vi "duplicates.vi"(11 "Array":string[](array[string])=["a", "b", "f", "e", "d"]) -> (3 "Array 2":string[](array[string]))   [LabVIEW 2014]
uses:
  Alphabet.ctl
  Counting.ctl
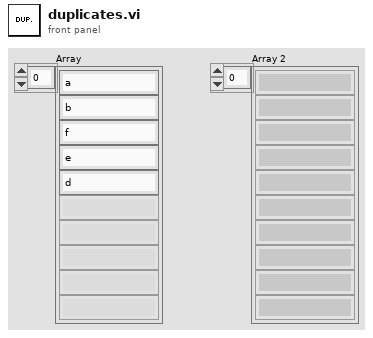
[diagram p1: front panel]
types:
  T1 = typedef "Counting.ctl" = cluster{"list":i32[], "a":i32}
  T2 = typedef "Alphabet.ctl" = enum16{"a", "b", "c", "d", "e", "f", "g", "h", "i", "j", "k", "l", "m", "n", "o", "p", "q", "r", "s", "t", "u", "v", "x", "y", "w", "z", "output"}
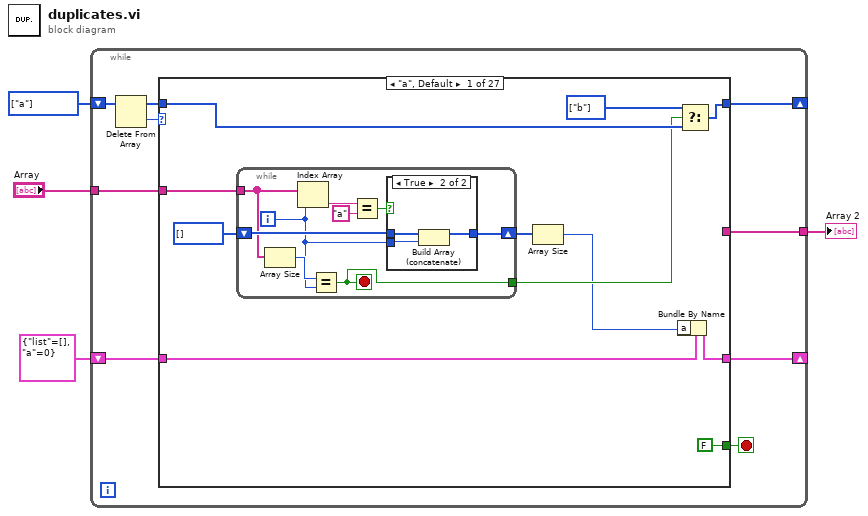
[diagram p0: block diagram]
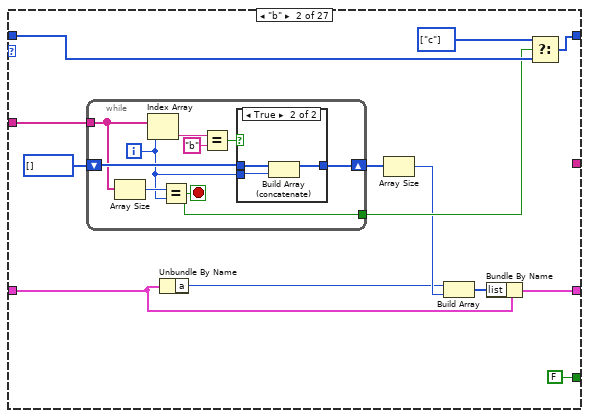
[diagram p3: hidden frame]
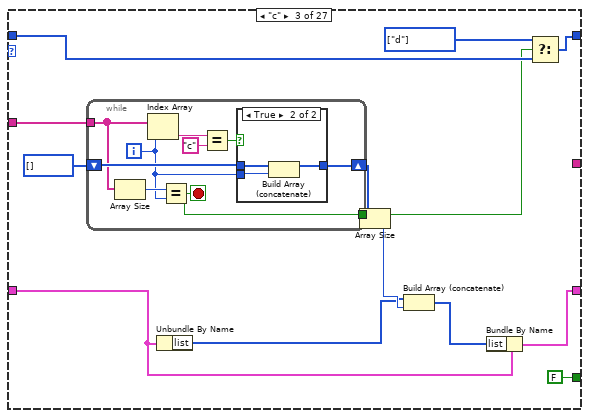
[diagram p5: hidden frame]
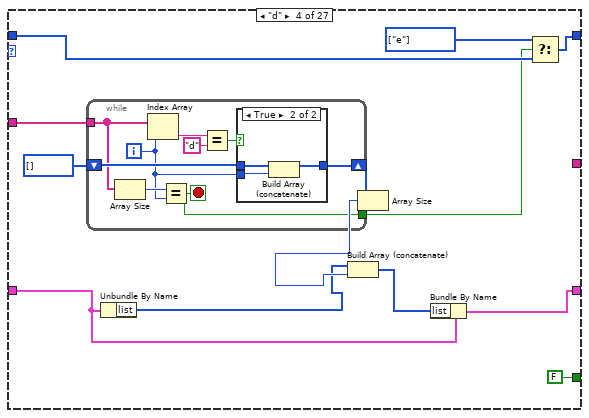
[diagram p7: hidden frame]
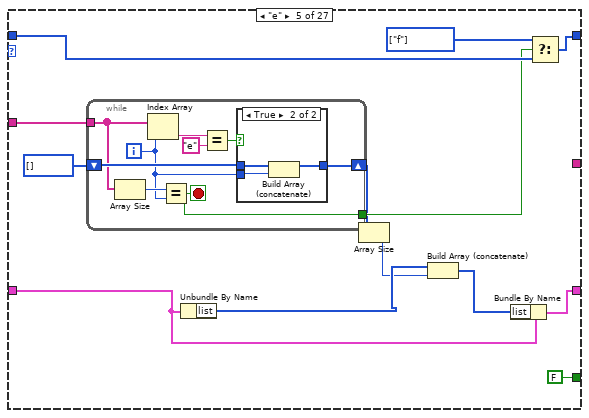
[diagram p9: hidden frame]
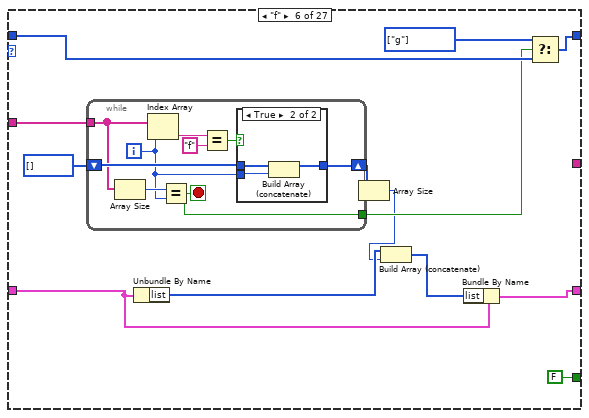
[diagram p11: hidden frame]
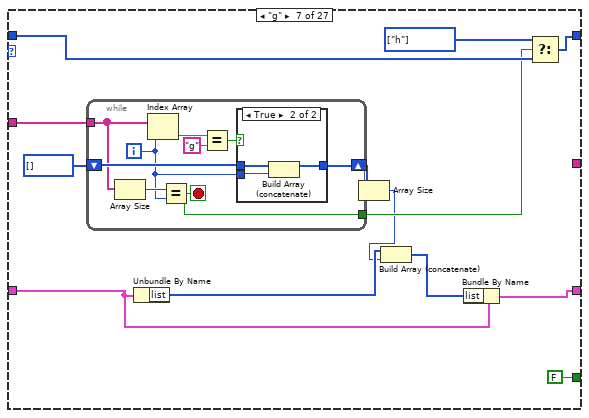
[diagram p13: hidden frame]
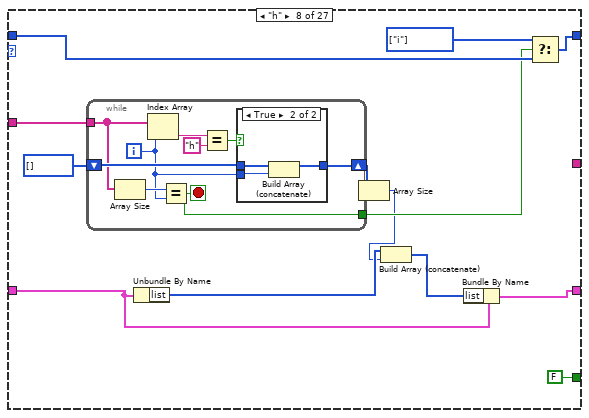
[diagram p15: hidden frame]
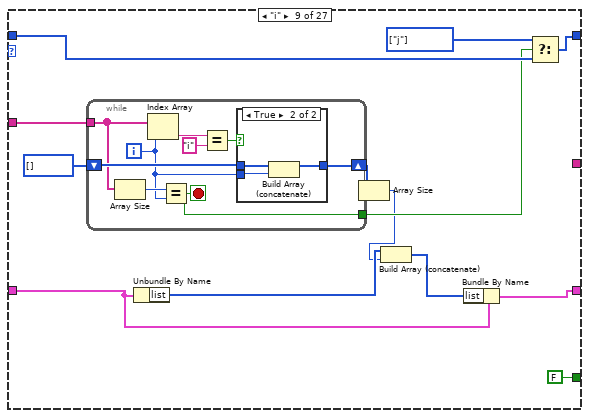
[diagram p17: hidden frame]
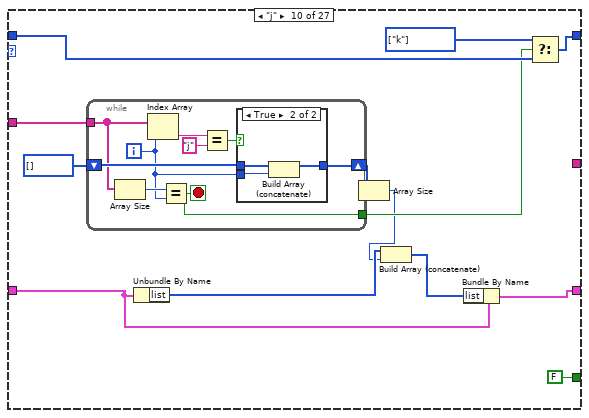
[diagram p19: hidden frame]
diagram:
  w4 = T2[] [enum."a"] items=["a", "b", "c", "d", "e", "f", "g", "h", "i", "j", "k", "l", "m", "n", "o", "p", "q", "r", "s", "t", "u", "v", "x", "y", "w", "z", "output"]
  n1 = while {
    shift-right: [w11] -> _
    shift-left: w4 -> [w13]
    tunnel: "Array" -> [w9]
    shift-right: [w6] -> _
    shift-left: T1 {"list"=[], "a"=0} -> [w7]
    tunnel: [w5] -> w1
    stop <- w8 stop-if-true
    n2 = Delete From Array(array=w13) -> (deleted portion=w12:T2, array with subset deleted=w10:T2[])  [unwired: 2 in]
    n3 = case shown="\"a\", Default" w12 {
      tunnel: [w21 w47 w73 w99 w125 w151 w177 w203 w229 w255 w281 w307 w333 w359 w385 w411 w437 w463 w489 w515 w541 w567 w593 w619 w645 w671 w690] -> w11
      tunnel: w10 -> [w23 w49 w75 w101 w127 w153 w179 w205 w231 w257 w283 w309 w335 w361 w387 w413 w439 w465 w491 w517 w543 w569 w595 w621 w647 w673 w690]
      tunnel: w9 -> [w24 w50 w76 w102 w128 w154 w180 w206 w232 w258 w284 w310 w336 w362 w388 w414 w440 w466 w492 w518 w544 w570 w596 w622 w648 w674 _]
      tunnel: [FALSE FALSE FALSE FALSE FALSE FALSE FALSE FALSE FALSE FALSE FALSE FALSE FALSE FALSE FALSE FALSE FALSE FALSE FALSE FALSE FALSE FALSE FALSE FALSE FALSE FALSE TRUE] -> w8
      tunnel: w7 -> [w16 w42 w68 w94 w118 w144 w170 w196 w222 w248 w274 w300 w326 w352 w378 w404 w430 w456 w482 w508 w534 w560 w586 w612 w638 w664 w692]
      tunnel: [w15 w41 w67 w93 w119 w145 w171 w197 w223 w249 w275 w301 w327 w353 w379 w405 w431 w457 w483 w509 w535 w561 w587 w613 w639 w665 w692] -> w6
      tunnel: [_ _ _ _ _ _ _ _ _ _ _ _ _ _ _ _ _ _ _ _ _ _ _ _ _ _ w688] -> w5
      frame "a", Default {
        w22 = T2[] [enum."b"] items=["a", "b", "c", "d", "e", "f", "g", "h", "i", "j", "k", "l", "m", "n", "o", "p", "q", "r", "s", "t", "u", "v", "x", "y", "w", "z", "output"]
        n4 = while {
          tunnel: w24 -> [w28]
          shift-right: [w29] -> w17
          shift-left: i32[] [] -> [w30]
          tunnel: [w25] -> w18
          i -> [w26]
          stop <- w25 stop-if-true
          n5 = Array Size(array=w28) -> (size(s)=w27:i32)
          n6 = Index Array(array=w28, index=w26) -> (element=w31:string)
          n7 = Equal?(x=w27, y=w26) -> (x = y?=w25:bool)
          n8 = Equal?(x=w31, y="a") -> (x = y?=w32:bool)
          n9 = case shown="True" w32 {
            tunnel: w26 -> [_ w37]
            tunnel: w30 -> [w34 w36]
            tunnel: [w34 w35] -> w29
            frame False {
            }
            frame True {
              n10 = Build Array (concatenate)(w36, w37) -> (w35:i32[])
            }
          }
        }
        n11 = Array Size(array=w17) -> (size(s)=w14:i32)
        n12 = Bundle By Name(cluster=w16, "a"=w14) -> (w15:T1)
        n13 = Select(t=w22, s=w18, f=w23) -> (s? t:f=w21:T2[])
      }
      frame "b" {
        w48 = T2[] [enum."c"] items=["a", "b", "c", "d", "e", "f", "g", "h", "i", "j", "k", "l", "m", "n", "o", "p", "q", "r", "s", "t", "u", "v", "x", "y", "w", "z", "output"]
        n14 = while {
          tunnel: w50 -> [w54]
          shift-right: [w55] -> w43
          shift-left: i32[] [] -> [w56]
          tunnel: [w51] -> w44
          i -> [w52]
          stop <- w51 stop-if-true
          n15 = Array Size(array=w54) -> (size(s)=w53:i32)
          n16 = Index Array(array=w54, index=w52) -> (element=w57:string)
          n17 = Equal?(x=w53, y=w52) -> (x = y?=w51:bool)
          n18 = Equal?(x=w57, y="b") -> (x = y?=w58:bool)
          n19 = case shown="True" w58 {
            tunnel: w52 -> [_ w63]
            tunnel: w56 -> [w60 w62]
            tunnel: [w60 w61] -> w55
            frame False {
            }
            frame True {
              n20 = Build Array (concatenate)(w62, w63) -> (w61:i32[])
            }
          }
        }
        n21 = Unbundle By Name(w42) -> ("a"=w38:i32)
        n22 = Array Size(array=w43) -> (size(s)=w39:i32)
        n23 = Build Array(w38, w39) -> (w40:i32[])
        n24 = Bundle By Name(cluster=w42, "list"=w40) -> (w41:T1)
        n25 = Select(t=w48, s=w44, f=w49) -> (s? t:f=w47:T2[])
      }
      frame "c" {
        w74 = T2[] [enum."d"] items=["a", "b", "c", "d", "e", "f", "g", "h", "i", "j", "k", "l", "m", "n", "o", "p", "q", "r", "s", "t", "u", "v", "x", "y", "w", "z", "output"]
        n26 = while {
          tunnel: w76 -> [w80]
          shift-right: [w81] -> w66
          shift-left: i32[] [] -> [w82]
          tunnel: [w77] -> w70
          i -> [w78]
          stop <- w77 stop-if-true
          n27 = Array Size(array=w80) -> (size(s)=w79:i32)
          n28 = Index Array(array=w80, index=w78) -> (element=w83:string)
          n29 = Equal?(x=w79, y=w78) -> (x = y?=w77:bool)
          n30 = Equal?(x=w83, y="c") -> (x = y?=w84:bool)
          n31 = case shown="True" w84 {
            tunnel: w78 -> [_ w89]
            tunnel: w82 -> [w86 w88]
            tunnel: [w86 w87] -> w81
            frame False {
            }
            frame True {
              n32 = Build Array (concatenate)(w88, w89) -> (w87:i32[])
            }
          }
        }
        n33 = Unbundle By Name(w68) -> ("list"=w64:i32[])
        n34 = Array Size(array=w66) -> (size(s)=w65:i32)
        n35 = Build Array (concatenate)(w64, w65) -> (w69:i32[])
        n36 = Bundle By Name(cluster=w68, "list"=w69) -> (w67:T1)
        n37 = Select(t=w74, s=w70, f=w75) -> (s? t:f=w73:T2[])
      }
      frame "d" {
        w100 = T2[] [enum."e"] items=["a", "b", "c", "d", "e", "f", "g", "h", "i", "j", "k", "l", "m", "n", "o", "p", "q", "r", "s", "t", "u", "v", "x", "y", "w", "z", "output"]
        n38 = while {
          tunnel: w102 -> [w106]
          shift-right: [w107] -> w92
          shift-left: i32[] [] -> [w108]
          tunnel: [w103] -> w96
          i -> [w104]
          stop <- w103 stop-if-true
          n39 = Array Size(array=w106) -> (size(s)=w105:i32)
          n40 = Index Array(array=w106, index=w104) -> (element=w109:string)
          n41 = Equal?(x=w105, y=w104) -> (x = y?=w103:bool)
          n42 = Equal?(x=w109, y="d") -> (x = y?=w110:bool)
          n43 = case shown="True" w110 {
            tunnel: w104 -> [_ w115]
            tunnel: w108 -> [w112 w114]
            tunnel: [w112 w113] -> w107
            frame False {
            }
            frame True {
              n44 = Build Array (concatenate)(w114, w115) -> (w113:i32[])
            }
          }
        }
        n45 = Unbundle By Name(w94) -> ("list"=w90:i32[])
        n46 = Array Size(array=w92) -> (size(s)=w91:i32)
        n47 = Build Array (concatenate)(w90, w91) -> (w95:i32[])
        n48 = Bundle By Name(cluster=w94, "list"=w95) -> (w93:T1)
        n49 = Select(t=w100, s=w96, f=w101) -> (s? t:f=w99:T2[])
      }
      frame "e" {
        w126 = T2[] [enum."f"] items=["a", "b", "c", "d", "e", "f", "g", "h", "i", "j", "k", "l", "m", "n", "o", "p", "q", "r", "s", "t", "u", "v", "x", "y", "w", "z", "output"]
        n50 = while {
          tunnel: w128 -> [w132]
          shift-right: [w133] -> w120
          shift-left: i32[] [] -> [w134]
          tunnel: [w129] -> w122
          i -> [w130]
          stop <- w129 stop-if-true
          n51 = Array Size(array=w132) -> (size(s)=w131:i32)
          n52 = Index Array(array=w132, index=w130) -> (element=w135:string)
          n53 = Equal?(x=w131, y=w130) -> (x = y?=w129:bool)
          n54 = Equal?(x=w135, y="e") -> (x = y?=w136:bool)
          n55 = case shown="True" w136 {
            tunnel: w130 -> [_ w141]
            tunnel: w134 -> [w138 w140]
            tunnel: [w138 w139] -> w133
            frame False {
            }
            frame True {
              n56 = Build Array (concatenate)(w140, w141) -> (w139:i32[])
            }
          }
        }
        n57 = Unbundle By Name(w118) -> ("list"=w117:i32[])
        n58 = Array Size(array=w120) -> (size(s)=w116:i32)
        n59 = Build Array (concatenate)(w117, w116) -> (w121:i32[])
        n60 = Bundle By Name(cluster=w118, "list"=w121) -> (w119:T1)
        n61 = Select(t=w126, s=w122, f=w127) -> (s? t:f=w125:T2[])
      }
      frame "f" {
        w152 = T2[] [enum."g"] items=["a", "b", "c", "d", "e", "f", "g", "h", "i", "j", "k", "l", "m", "n", "o", "p", "q", "r", "s", "t", "u", "v", "x", "y", "w", "z", "output"]
        n62 = while {
          tunnel: w154 -> [w158]
          shift-right: [w159] -> w146
          shift-left: i32[] [] -> [w160]
          tunnel: [w155] -> w148
          i -> [w156]
          stop <- w155 stop-if-true
          n63 = Array Size(array=w158) -> (size(s)=w157:i32)
          n64 = Index Array(array=w158, index=w156) -> (element=w161:string)
          n65 = Equal?(x=w157, y=w156) -> (x = y?=w155:bool)
          n66 = Equal?(x=w161, y="f") -> (x = y?=w162:bool)
          n67 = case shown="True" w162 {
            tunnel: w156 -> [_ w167]
            tunnel: w160 -> [w164 w166]
            tunnel: [w164 w165] -> w159
            frame False {
            }
            frame True {
              n68 = Build Array (concatenate)(w166, w167) -> (w165:i32[])
            }
          }
        }
        n69 = Unbundle By Name(w144) -> ("list"=w143:i32[])
        n70 = Array Size(array=w146) -> (size(s)=w142:i32)
        n71 = Build Array (concatenate)(w143, w142) -> (w147:i32[])
        n72 = Bundle By Name(cluster=w144, "list"=w147) -> (w145:T1)
        n73 = Select(t=w152, s=w148, f=w153) -> (s? t:f=w151:T2[])
      }
      frame "g" {
        w178 = T2[] [enum."h"] items=["a", "b", "c", "d", "e", "f", "g", "h", "i", "j", "k", "l", "m", "n", "o", "p", "q", "r", "s", "t", "u", "v", "x", "y", "w", "z", "output"]
        n74 = while {
          tunnel: w180 -> [w184]
          shift-right: [w185] -> w172
          shift-left: i32[] [] -> [w186]
          tunnel: [w181] -> w174
          i -> [w182]
          stop <- w181 stop-if-true
          n75 = Array Size(array=w184) -> (size(s)=w183:i32)
          n76 = Index Array(array=w184, index=w182) -> (element=w187:string)
          n77 = Equal?(x=w183, y=w182) -> (x = y?=w181:bool)
          n78 = Equal?(x=w187, y="g") -> (x = y?=w188:bool)
          n79 = case shown="True" w188 {
            tunnel: w182 -> [_ w193]
            tunnel: w186 -> [w190 w192]
            tunnel: [w190 w191] -> w185
            frame False {
            }
            frame True {
              n80 = Build Array (concatenate)(w192, w193) -> (w191:i32[])
            }
          }
        }
        n81 = Unbundle By Name(w170) -> ("list"=w169:i32[])
        n82 = Array Size(array=w172) -> (size(s)=w168:i32)
        n83 = Build Array (concatenate)(w169, w168) -> (w173:i32[])
        n84 = Bundle By Name(cluster=w170, "list"=w173) -> (w171:T1)
        n85 = Select(t=w178, s=w174, f=w179) -> (s? t:f=w177:T2[])
      }
      frame "h" {
        w204 = T2[] [enum."i"] items=["a", "b", "c", "d", "e", "f", "g", "h", "i", "j", "k", "l", "m", "n", "o", "p", "q", "r", "s", "t", "u", "v", "x", "y", "w", "z", "output"]
        n86 = while {
          tunnel: w206 -> [w210]
          shift-right: [w211] -> w198
          shift-left: i32[] [] -> [w212]
          tunnel: [w207] -> w200
          i -> [w208]
          stop <- w207 stop-if-true
          n87 = Array Size(array=w210) -> (size(s)=w209:i32)
          n88 = Index Array(array=w210, index=w208) -> (element=w213:string)
          n89 = Equal?(x=w209, y=w208) -> (x = y?=w207:bool)
          n90 = Equal?(x=w213, y="h") -> (x = y?=w214:bool)
          n91 = case shown="True" w214 {
            tunnel: w208 -> [_ w219]
            tunnel: w212 -> [w216 w218]
            tunnel: [w216 w217] -> w211
            frame False {
            }
            frame True {
              n92 = Build Array (concatenate)(w218, w219) -> (w217:i32[])
            }
          }
        }
        n93 = Unbundle By Name(w196) -> ("list"=w195:i32[])
        n94 = Array Size(array=w198) -> (size(s)=w194:i32)
        n95 = Build Array (concatenate)(w195, w194) -> (w199:i32[])
        n96 = Bundle By Name(cluster=w196, "list"=w199) -> (w197:T1)
        n97 = Select(t=w204, s=w200, f=w205) -> (s? t:f=w203:T2[])
      }
      frame "i" {
        w230 = T2[] [enum."j"] items=["a", "b", "c", "d", "e", "f", "g", "h", "i", "j", "k", "l", "m", "n", "o", "p", "q", "r", "s", "t", "u", "v", "x", "y", "w", "z", "output"]
        n98 = while {
          tunnel: w232 -> [w236]
          shift-right: [w237] -> w224
          shift-left: i32[] [] -> [w238]
          tunnel: [w233] -> w226
          i -> [w234]
          stop <- w233 stop-if-true
          n99 = Array Size(array=w236) -> (size(s)=w235:i32)
          n100 = Index Array(array=w236, index=w234) -> (element=w239:string)
          n101 = Equal?(x=w235, y=w234) -> (x = y?=w233:bool)
          n102 = Equal?(x=w239, y="i") -> (x = y?=w240:bool)
          n103 = case shown="True" w240 {
            tunnel: w234 -> [_ w245]
            tunnel: w238 -> [w242 w244]
            tunnel: [w242 w243] -> w237
            frame False {
            }
            frame True {
              n104 = Build Array (concatenate)(w244, w245) -> (w243:i32[])
            }
          }
        }
        n105 = Unbundle By Name(w222) -> ("list"=w221:i32[])
        n106 = Array Size(array=w224) -> (size(s)=w220:i32)
        n107 = Build Array (concatenate)(w221, w220) -> (w225:i32[])
        n108 = Bundle By Name(cluster=w222, "list"=w225) -> (w223:T1)
        n109 = Select(t=w230, s=w226, f=w231) -> (s? t:f=w229:T2[])
      }
      frame "j" {
        w256 = T2[] [enum."k"] items=["a", "b", "c", "d", "e", "f", "g", "h", "i", "j", "k", "l", "m", "n", "o", "p", "q", "r", "s", "t", "u", "v", "x", "y", "w", "z", "output"]
        n110 = while {
          tunnel: w258 -> [w262]
          shift-right: [w263] -> w250
          shift-left: i32[] [] -> [w264]
          tunnel: [w259] -> w252
          i -> [w260]
          stop <- w259 stop-if-true
          n111 = Array Size(array=w262) -> (size(s)=w261:i32)
          n112 = Index Array(array=w262, index=w260) -> (element=w265:string)
          n113 = Equal?(x=w261, y=w260) -> (x = y?=w259:bool)
          n114 = Equal?(x=w265, y="j") -> (x = y?=w266:bool)
          n115 = case shown="True" w266 {
            tunnel: w260 -> [_ w271]
            tunnel: w264 -> [w268 w270]
            tunnel: [w268 w269] -> w263
            frame False {
            }
            frame True {
              n116 = Build Array (concatenate)(w270, w271) -> (w269:i32[])
            }
          }
        }
        n117 = Unbundle By Name(w248) -> ("list"=w247:i32[])
        n118 = Array Size(array=w250) -> (size(s)=w246:i32)
        n119 = Build Array (concatenate)(w247, w246) -> (w251:i32[])
        n120 = Bundle By Name(cluster=w248, "list"=w251) -> (w249:T1)
        n121 = Select(t=w256, s=w252, f=w257) -> (s? t:f=w255:T2[])
      }
      frame "k" {
        w282 = T2[] [enum."l"] items=["a", "b", "c", "d", "e", "f", "g", "h", "i", "j", "k", "l", "m", "n", "o", "p", "q", "r", "s", "t", "u", "v", "x", "y", "w", "z", "output"]
        n122 = while {
          tunnel: w284 -> [w288]
          shift-right: [w289] -> w276
          shift-left: i32[] [] -> [w290]
          tunnel: [w285] -> w278
          i -> [w286]
          stop <- w285 stop-if-true
          n123 = Array Size(array=w288) -> (size(s)=w287:i32)
          n124 = Index Array(array=w288, index=w286) -> (element=w291:string)
          n125 = Equal?(x=w287, y=w286) -> (x = y?=w285:bool)
          n126 = Equal?(x=w291, y="k") -> (x = y?=w292:bool)
          n127 = case shown="True" w292 {
            tunnel: w286 -> [_ w297]
            tunnel: w290 -> [w294 w296]
            tunnel: [w294 w295] -> w289
            frame False {
            }
            frame True {
              n128 = Build Array (concatenate)(w296, w297) -> (w295:i32[])
            }
          }
        }
        n129 = Unbundle By Name(w274) -> ("list"=w273:i32[])
        n130 = Array Size(array=w276) -> (size(s)=w272:i32)
        n131 = Build Array (concatenate)(w273, w272) -> (w277:i32[])
        n132 = Bundle By Name(cluster=w274, "list"=w277) -> (w275:T1)
        n133 = Select(t=w282, s=w278, f=w283) -> (s? t:f=w281:T2[])
      }
      frame "l" {
        w308 = T2[] [enum."m"] items=["a", "b", "c", "d", "e", "f", "g", "h", "i", "j", "k", "l", "m", "n", "o", "p", "q", "r", "s", "t", "u", "v", "x", "y", "w", "z", "output"]
        n134 = while {
          tunnel: w310 -> [w314]
          shift-right: [w315] -> w302
          shift-left: i32[] [] -> [w316]
          tunnel: [w311] -> w304
          i -> [w312]
          stop <- w311 stop-if-true
          n135 = Array Size(array=w314) -> (size(s)=w313:i32)
          n136 = Index Array(array=w314, index=w312) -> (element=w317:string)
          n137 = Equal?(x=w313, y=w312) -> (x = y?=w311:bool)
          n138 = Equal?(x=w317, y="l") -> (x = y?=w318:bool)
          n139 = case shown="True" w318 {
            tunnel: w312 -> [_ w323]
            tunnel: w316 -> [w320 w322]
            tunnel: [w320 w321] -> w315
            frame False {
            }
            frame True {
              n140 = Build Array (concatenate)(w322, w323) -> (w321:i32[])
            }
          }
        }
        n141 = Unbundle By Name(w300) -> ("list"=w299:i32[])
        n142 = Array Size(array=w302) -> (size(s)=w298:i32)
        n143 = Build Array (concatenate)(w299, w298) -> (w303:i32[])
        n144 = Bundle By Name(cluster=w300, "list"=w303) -> (w301:T1)
        n145 = Select(t=w308, s=w304, f=w309) -> (s? t:f=w307:T2[])
      }
      frame "m" {
        w334 = T2[] [enum."n"] items=["a", "b", "c", "d", "e", "f", "g", "h", "i", "j", "k", "l", "m", "n", "o", "p", "q", "r", "s", "t", "u", "v", "x", "y", "w", "z", "output"]
        n146 = while {
          tunnel: w336 -> [w340]
          shift-right: [w341] -> w328
          shift-left: i32[] [] -> [w342]
          tunnel: [w337] -> w330
          i -> [w338]
          stop <- w337 stop-if-true
          n147 = Array Size(array=w340) -> (size(s)=w339:i32)
          n148 = Index Array(array=w340, index=w338) -> (element=w343:string)
          n149 = Equal?(x=w339, y=w338) -> (x = y?=w337:bool)
          n150 = Equal?(x=w343, y="m") -> (x = y?=w344:bool)
          n151 = case shown="True" w344 {
            tunnel: w338 -> [_ w349]
            tunnel: w342 -> [w346 w348]
            tunnel: [w346 w347] -> w341
            frame False {
            }
            frame True {
              n152 = Build Array (concatenate)(w348, w349) -> (w347:i32[])
            }
          }
        }
        n153 = Unbundle By Name(w326) -> ("list"=w325:i32[])
        n154 = Array Size(array=w328) -> (size(s)=w324:i32)
        n155 = Build Array (concatenate)(w325, w324) -> (w329:i32[])
        n156 = Bundle By Name(cluster=w326, "list"=w329) -> (w327:T1)
        n157 = Select(t=w334, s=w330, f=w335) -> (s? t:f=w333:T2[])
      }
      frame "n" {
        w360 = T2[] [enum."o"] items=["a", "b", "c", "d", "e", "f", "g", "h", "i", "j", "k", "l", "m", "n", "o", "p", "q", "r", "s", "t", "u", "v", "x", "y", "w", "z", "output"]
        n158 = while {
          tunnel: w362 -> [w366]
          shift-right: [w367] -> w354
          shift-left: i32[] [] -> [w368]
          tunnel: [w363] -> w356
          i -> [w364]
          stop <- w363 stop-if-true
          n159 = Array Size(array=w366) -> (size(s)=w365:i32)
          n160 = Index Array(array=w366, index=w364) -> (element=w369:string)
          n161 = Equal?(x=w365, y=w364) -> (x = y?=w363:bool)
          n162 = Equal?(x=w369, y="n") -> (x = y?=w370:bool)
          n163 = case shown="True" w370 {
            tunnel: w364 -> [_ w375]
            tunnel: w368 -> [w372 w374]
            tunnel: [w372 w373] -> w367
            frame False {
            }
            frame True {
              n164 = Build Array (concatenate)(w374, w375) -> (w373:i32[])
            }
          }
        }
        n165 = Unbundle By Name(w352) -> ("list"=w351:i32[])
        n166 = Array Size(array=w354) -> (size(s)=w350:i32)
        n167 = Build Array (concatenate)(w351, w350) -> (w355:i32[])
        n168 = Bundle By Name(cluster=w352, "list"=w355) -> (w353:T1)
        n169 = Select(t=w360, s=w356, f=w361) -> (s? t:f=w359:T2[])
      }
      frame "o" {
        w386 = T2[] [enum."p"] items=["a", "b", "c", "d", "e", "f", "g", "h", "i", "j", "k", "l", "m", "n", "o", "p", "q", "r", "s", "t", "u", "v", "x", "y", "w", "z", "output"]
        n170 = while {
          tunnel: w388 -> [w392]
          shift-right: [w393] -> w380
          shift-left: i32[] [] -> [w394]
          tunnel: [w389] -> w382
          i -> [w390]
          stop <- w389 stop-if-true
          n171 = Array Size(array=w392) -> (size(s)=w391:i32)
          n172 = Index Array(array=w392, index=w390) -> (element=w395:string)
          n173 = Equal?(x=w391, y=w390) -> (x = y?=w389:bool)
          n174 = Equal?(x=w395, y="o") -> (x = y?=w396:bool)
          n175 = case shown="True" w396 {
            tunnel: w390 -> [_ w401]
            tunnel: w394 -> [w398 w400]
            tunnel: [w398 w399] -> w393
            frame False {
            }
            frame True {
              n176 = Build Array (concatenate)(w400, w401) -> (w399:i32[])
            }
          }
        }
        n177 = Unbundle By Name(w378) -> ("list"=w377:i32[])
        n178 = Array Size(array=w380) -> (size(s)=w376:i32)
        n179 = Build Array (concatenate)(w377, w376) -> (w381:i32[])
        n180 = Bundle By Name(cluster=w378, "list"=w381) -> (w379:T1)
        n181 = Select(t=w386, s=w382, f=w387) -> (s? t:f=w385:T2[])
      }
      frame "p" {
        w412 = T2[] [enum."q"] items=["a", "b", "c", "d", "e", "f", "g", "h", "i", "j", "k", "l", "m", "n", "o", "p", "q", "r", "s", "t", "u", "v", "x", "y", "w", "z", "output"]
        n182 = while {
          tunnel: w414 -> [w418]
          shift-right: [w419] -> w406
          shift-left: i32[] [] -> [w420]
          tunnel: [w415] -> w408
          i -> [w416]
          stop <- w415 stop-if-true
          n183 = Array Size(array=w418) -> (size(s)=w417:i32)
          n184 = Index Array(array=w418, index=w416) -> (element=w421:string)
          n185 = Equal?(x=w417, y=w416) -> (x = y?=w415:bool)
          n186 = Equal?(x=w421, y="p") -> (x = y?=w422:bool)
          n187 = case shown="True" w422 {
            tunnel: w416 -> [_ w427]
            tunnel: w420 -> [w424 w426]
            tunnel: [w424 w425] -> w419
            frame False {
            }
            frame True {
              n188 = Build Array (concatenate)(w426, w427) -> (w425:i32[])
            }
          }
        }
        n189 = Unbundle By Name(w404) -> ("list"=w403:i32[])
        n190 = Array Size(array=w406) -> (size(s)=w402:i32)
        n191 = Build Array (concatenate)(w403, w402) -> (w407:i32[])
        n192 = Bundle By Name(cluster=w404, "list"=w407) -> (w405:T1)
        n193 = Select(t=w412, s=w408, f=w413) -> (s? t:f=w411:T2[])
      }
      frame "q" {
        w438 = T2[] [enum."r"] items=["a", "b", "c", "d", "e", "f", "g", "h", "i", "j", "k", "l", "m", "n", "o", "p", "q", "r", "s", "t", "u", "v", "x", "y", "w", "z", "output"]
        n194 = while {
          tunnel: w440 -> [w444]
          shift-right: [w445] -> w432
          shift-left: i32[] [] -> [w446]
          tunnel: [w441] -> w434
          i -> [w442]
          stop <- w441 stop-if-true
          n195 = Array Size(array=w444) -> (size(s)=w443:i32)
          n196 = Index Array(array=w444, index=w442) -> (element=w447:string)
          n197 = Equal?(x=w443, y=w442) -> (x = y?=w441:bool)
          n198 = Equal?(x=w447, y="q") -> (x = y?=w448:bool)
          n199 = case shown="True" w448 {
            tunnel: w442 -> [_ w453]
            tunnel: w446 -> [w450 w452]
            tunnel: [w450 w451] -> w445
            frame False {
            }
            frame True {
              n200 = Build Array (concatenate)(w452, w453) -> (w451:i32[])
            }
          }
        }
        n201 = Unbundle By Name(w430) -> ("list"=w429:i32[])
        n202 = Array Size(array=w432) -> (size(s)=w428:i32)
        n203 = Build Array (concatenate)(w429, w428) -> (w433:i32[])
        n204 = Bundle By Name(cluster=w430, "list"=w433) -> (w431:T1)
        n205 = Select(t=w438, s=w434, f=w439) -> (s? t:f=w437:T2[])
      }
      frame "r" {
        w464 = T2[] [enum."s"] items=["a", "b", "c", "d", "e", "f", "g", "h", "i", "j", "k", "l", "m", "n", "o", "p", "q", "r", "s", "t", "u", "v", "x", "y", "w", "z", "output"]
        n206 = while {
          tunnel: w466 -> [w470]
          shift-right: [w471] -> w458
          shift-left: i32[] [] -> [w472]
          tunnel: [w467] -> w460
          i -> [w468]
          stop <- w467 stop-if-true
          n207 = Array Size(array=w470) -> (size(s)=w469:i32)
          n208 = Index Array(array=w470, index=w468) -> (element=w473:string)
          n209 = Equal?(x=w469, y=w468) -> (x = y?=w467:bool)
          n210 = Equal?(x=w473, y="r") -> (x = y?=w474:bool)
          n211 = case shown="True" w474 {
            tunnel: w468 -> [_ w479]
            tunnel: w472 -> [w476 w478]
            tunnel: [w476 w477] -> w471
            frame False {
            }
            frame True {
              n212 = Build Array (concatenate)(w478, w479) -> (w477:i32[])
            }
          }
        }
        n213 = Unbundle By Name(w456) -> ("list"=w455:i32[])
        n214 = Array Size(array=w458) -> (size(s)=w454:i32)
        n215 = Build Array (concatenate)(w455, w454) -> (w459:i32[])
        n216 = Bundle By Name(cluster=w456, "list"=w459) -> (w457:T1)
        n217 = Select(t=w464, s=w460, f=w465) -> (s? t:f=w463:T2[])
      }
      frame "s" {
        w490 = T2[] [enum."t"] items=["a", "b", "c", "d", "e", "f", "g", "h", "i", "j", "k", "l", "m", "n", "o", "p", "q", "r", "s", "t", "u", "v", "x", "y", "w", "z", "output"]
        n218 = while {
          tunnel: w492 -> [w496]
          shift-right: [w497] -> w484
          shift-left: i32[] [] -> [w498]
          tunnel: [w493] -> w486
          i -> [w494]
          stop <- w493 stop-if-true
          n219 = Array Size(array=w496) -> (size(s)=w495:i32)
          n220 = Index Array(array=w496, index=w494) -> (element=w499:string)
          n221 = Equal?(x=w495, y=w494) -> (x = y?=w493:bool)
          n222 = Equal?(x=w499, y="s") -> (x = y?=w500:bool)
          n223 = case shown="True" w500 {
            tunnel: w494 -> [_ w505]
            tunnel: w498 -> [w502 w504]
            tunnel: [w502 w503] -> w497
            frame False {
            }
            frame True {
              n224 = Build Array (concatenate)(w504, w505) -> (w503:i32[])
            }
          }
        }
        n225 = Unbundle By Name(w482) -> ("list"=w481:i32[])
        n226 = Array Size(array=w484) -> (size(s)=w480:i32)
        n227 = Build Array (concatenate)(w481, w480) -> (w485:i32[])
        n228 = Bundle By Name(cluster=w482, "list"=w485) -> (w483:T1)
        n229 = Select(t=w490, s=w486, f=w491) -> (s? t:f=w489:T2[])
      }
      frame "t" {
        w516 = T2[] [enum."u"] items=["a", "b", "c", "d", "e", "f", "g", "h", "i", "j", "k", "l", "m", "n", "o", "p", "q", "r", "s", "t", "u", "v", "x", "y", "w", "z", "output"]
        n230 = while {
          tunnel: w518 -> [w522]
          shift-right: [w523] -> w510
          shift-left: i32[] [] -> [w524]
          tunnel: [w519] -> w512
          i -> [w520]
          stop <- w519 stop-if-true
          n231 = Array Size(array=w522) -> (size(s)=w521:i32)
          n232 = Index Array(array=w522, index=w520) -> (element=w525:string)
          n233 = Equal?(x=w521, y=w520) -> (x = y?=w519:bool)
          n234 = Equal?(x=w525, y="t") -> (x = y?=w526:bool)
          n235 = case shown="True" w526 {
            tunnel: w520 -> [_ w531]
            tunnel: w524 -> [w528 w530]
            tunnel: [w528 w529] -> w523
            frame False {
            }
            frame True {
              n236 = Build Array (concatenate)(w530, w531) -> (w529:i32[])
            }
          }
        }
        n237 = Unbundle By Name(w508) -> ("list"=w507:i32[])
        n238 = Array Size(array=w510) -> (size(s)=w506:i32)
        n239 = Build Array (concatenate)(w507, w506) -> (w511:i32[])
        n240 = Bundle By Name(cluster=w508, "list"=w511) -> (w509:T1)
        n241 = Select(t=w516, s=w512, f=w517) -> (s? t:f=w515:T2[])
      }
      frame "u" {
        w542 = T2[] [enum."v"] items=["a", "b", "c", "d", "e", "f", "g", "h", "i", "j", "k", "l", "m", "n", "o", "p", "q", "r", "s", "t", "u", "v", "x", "y", "w", "z", "output"]
        n242 = while {
          tunnel: w544 -> [w548]
          shift-right: [w549] -> w536
          shift-left: i32[] [] -> [w550]
          tunnel: [w545] -> w538
          i -> [w546]
          stop <- w545 stop-if-true
          n243 = Array Size(array=w548) -> (size(s)=w547:i32)
          n244 = Index Array(array=w548, index=w546) -> (element=w551:string)
          n245 = Equal?(x=w547, y=w546) -> (x = y?=w545:bool)
          n246 = Equal?(x=w551, y="u") -> (x = y?=w552:bool)
          n247 = case shown="True" w552 {
            tunnel: w546 -> [_ w557]
            tunnel: w550 -> [w554 w556]
            tunnel: [w554 w555] -> w549
            frame False {
            }
            frame True {
              n248 = Build Array (concatenate)(w556, w557) -> (w555:i32[])
            }
          }
        }
        n249 = Unbundle By Name(w534) -> ("list"=w533:i32[])
        n250 = Array Size(array=w536) -> (size(s)=w532:i32)
        n251 = Build Array (concatenate)(w533, w532) -> (w537:i32[])
        n252 = Bundle By Name(cluster=w534, "list"=w537) -> (w535:T1)
        n253 = Select(t=w542, s=w538, f=w543) -> (s? t:f=w541:T2[])
      }
      frame "v" {
        w568 = T2[] [enum."x"] items=["a", "b", "c", "d", "e", "f", "g", "h", "i", "j", "k", "l", "m", "n", "o", "p", "q", "r", "s", "t", "u", "v", "x", "y", "w", "z", "output"]
        n254 = while {
          tunnel: w570 -> [w574]
          shift-right: [w575] -> w562
          shift-left: i32[] [] -> [w576]
          tunnel: [w571] -> w564
          i -> [w572]
          stop <- w571 stop-if-true
          n255 = Array Size(array=w574) -> (size(s)=w573:i32)
          n256 = Index Array(array=w574, index=w572) -> (element=w577:string)
          n257 = Equal?(x=w573, y=w572) -> (x = y?=w571:bool)
          n258 = Equal?(x=w577, y="v") -> (x = y?=w578:bool)
          n259 = case shown="True" w578 {
            tunnel: w572 -> [_ w583]
            tunnel: w576 -> [w580 w582]
            tunnel: [w580 w581] -> w575
            frame False {
            }
            frame True {
              n260 = Build Array (concatenate)(w582, w583) -> (w581:i32[])
            }
          }
        }
        n261 = Unbundle By Name(w560) -> ("list"=w559:i32[])
        n262 = Array Size(array=w562) -> (size(s)=w558:i32)
        n263 = Build Array (concatenate)(w559, w558) -> (w563:i32[])
        n264 = Bundle By Name(cluster=w560, "list"=w563) -> (w561:T1)
        n265 = Select(t=w568, s=w564, f=w569) -> (s? t:f=w567:T2[])
      }
      frame "x" {
        w594 = T2[] [enum."y"] items=["a", "b", "c", "d", "e", "f", "g", "h", "i", "j", "k", "l", "m", "n", "o", "p", "q", "r", "s", "t", "u", "v", "x", "y", "w", "z", "output"]
        n266 = while {
          tunnel: w596 -> [w600]
          shift-right: [w601] -> w588
          shift-left: i32[] [] -> [w602]
          tunnel: [w597] -> w590
          i -> [w598]
          stop <- w597 stop-if-true
          n267 = Array Size(array=w600) -> (size(s)=w599:i32)
          n268 = Index Array(array=w600, index=w598) -> (element=w603:string)
          n269 = Equal?(x=w599, y=w598) -> (x = y?=w597:bool)
          n270 = Equal?(x=w603, y="x") -> (x = y?=w604:bool)
          n271 = case shown="True" w604 {
            tunnel: w598 -> [_ w609]
            tunnel: w602 -> [w606 w608]
            tunnel: [w606 w607] -> w601
            frame False {
            }
            frame True {
              n272 = Build Array (concatenate)(w608, w609) -> (w607:i32[])
            }
          }
        }
        n273 = Unbundle By Name(w586) -> ("list"=w585:i32[])
        n274 = Array Size(array=w588) -> (size(s)=w584:i32)
        n275 = Build Array (concatenate)(w585, w584) -> (w589:i32[])
        n276 = Bundle By Name(cluster=w586, "list"=w589) -> (w587:T1)
        n277 = Select(t=w594, s=w590, f=w595) -> (s? t:f=w593:T2[])
      }
      frame "y" {
        w620 = T2[] [enum."w"] items=["a", "b", "c", "d", "e", "f", "g", "h", "i", "j", "k", "l", "m", "n", "o", "p", "q", "r", "s", "t", "u", "v", "x", "y", "w", "z", "output"]
        n278 = while {
          tunnel: w622 -> [w626]
          shift-right: [w627] -> w614
          shift-left: i32[] [] -> [w628]
          tunnel: [w623] -> w616
          i -> [w624]
          stop <- w623 stop-if-true
          n279 = Array Size(array=w626) -> (size(s)=w625:i32)
          n280 = Index Array(array=w626, index=w624) -> (element=w629:string)
          n281 = Equal?(x=w625, y=w624) -> (x = y?=w623:bool)
          n282 = Equal?(x=w629, y="y") -> (x = y?=w630:bool)
          n283 = case shown="True" w630 {
            tunnel: w624 -> [_ w635]
            tunnel: w628 -> [w632 w634]
            tunnel: [w632 w633] -> w627
            frame False {
            }
            frame True {
              n284 = Build Array (concatenate)(w634, w635) -> (w633:i32[])
            }
          }
        }
        n285 = Unbundle By Name(w612) -> ("list"=w611:i32[])
        n286 = Array Size(array=w614) -> (size(s)=w610:i32)
        n287 = Build Array (concatenate)(w611, w610) -> (w615:i32[])
        n288 = Bundle By Name(cluster=w612, "list"=w615) -> (w613:T1)
        n289 = Select(t=w620, s=w616, f=w621) -> (s? t:f=w619:T2[])
      }
      frame "w" {
        w646 = T2[] [enum."z"] items=["a", "b", "c", "d", "e", "f", "g", "h", "i", "j", "k", "l", "m", "n", "o", "p", "q", "r", "s", "t", "u", "v", "x", "y", "w", "z", "output"]
        n290 = while {
          tunnel: w648 -> [w652]
          shift-right: [w653] -> w640
          shift-left: i32[] [] -> [w654]
          tunnel: [w649] -> w642
          i -> [w650]
          stop <- w649 stop-if-true
          n291 = Array Size(array=w652) -> (size(s)=w651:i32)
          n292 = Index Array(array=w652, index=w650) -> (element=w655:string)
          n293 = Equal?(x=w651, y=w650) -> (x = y?=w649:bool)
          n294 = Equal?(x=w655, y="w") -> (x = y?=w656:bool)
          n295 = case shown="True" w656 {
            tunnel: w650 -> [_ w661]
            tunnel: w654 -> [w658 w660]
            tunnel: [w658 w659] -> w653
            frame False {
            }
            frame True {
              n296 = Build Array (concatenate)(w660, w661) -> (w659:i32[])
            }
          }
        }
        n297 = Unbundle By Name(w638) -> ("list"=w637:i32[])
        n298 = Array Size(array=w640) -> (size(s)=w636:i32)
        n299 = Build Array (concatenate)(w637, w636) -> (w641:i32[])
        n300 = Bundle By Name(cluster=w638, "list"=w641) -> (w639:T1)
        n301 = Select(t=w646, s=w642, f=w647) -> (s? t:f=w645:T2[])
      }
      frame "z" {
        w672 = T2[] [enum."output"] items=["a", "b", "c", "d", "e", "f", "g", "h", "i", "j", "k", "l", "m", "n", "o", "p", "q", "r", "s", "t", "u", "v", "x", "y", "w", "z", "output"]
        n302 = while {
          tunnel: w674 -> [w678]
          shift-right: [w679] -> w666
          shift-left: i32[] [] -> [w680]
          tunnel: [w675] -> w668
          i -> [w676]
          stop <- w675 stop-if-true
          n303 = Array Size(array=w678) -> (size(s)=w677:i32)
          n304 = Index Array(array=w678, index=w676) -> (element=w681:string)
          n305 = Equal?(x=w677, y=w676) -> (x = y?=w675:bool)
          n306 = Equal?(x=w681, y="z") -> (x = y?=w682:bool)
          n307 = case shown="True" w682 {
            tunnel: w676 -> [_ w687]
            tunnel: w680 -> [w684 w686]
            tunnel: [w684 w685] -> w679
            frame False {
            }
            frame True {
              n308 = Build Array (concatenate)(w686, w687) -> (w685:i32[])
            }
          }
        }
        n309 = Unbundle By Name(w664) -> ("list"=w663:i32[])
        n310 = Array Size(array=w666) -> (size(s)=w662:i32)
        n311 = Build Array (concatenate)(w663, w662) -> (w667:i32[])
        n312 = Bundle By Name(cluster=w664, "list"=w667) -> (w665:T1)
        n313 = Select(t=w672, s=w668, f=w673) -> (s? t:f=w671:T2[])
      }
      frame "output" {
        n314 = Unbundle By Name(w692) -> ("list"=w694:i32[])
        n315 = while {
          tunnel: w694 -> [w701]
          shift-right: [w702] -> w688
          shift-left: string[] [] -> [w703]
          tunnel: string[] ["a", "b", "c", "d", "e", "f", "g", "h", "i", "j", "k", "l", "m", "n", "o", "p", "q", "r", "s", "t", "u", "v", "x", "y", "w", "z"] -> [w698]
          i -> [w697]
          stop <- w699 stop-if-true
          n316 = Index Array(array=w698, index=w697) -> (element=w696:string)
          n317 = Index Array(array=w701, index=w697) -> (element=w695:i32)
          n318 = Array Size(array=w701) -> (size(s)=w700:i32)
          n319 = case shown="\"0\", Default" w696 {
            tunnel: w703 -> [w704 w708 w715 w723 w731 w739 w747 w755 w763 w771 w779 w787 w795 w803 w811 w819 w827 w835 w843 w851 w859 w867 w875 w883 w891 w899 w907]
            tunnel: [w704 w707 w714 w722 w730 w738 w746 w754 w762 w770 w778 w786 w794 w802 w810 w818 w826 w834 w842 w850 w858 w866 w874 w882 w890 w898 w906] -> w702
            tunnel: w695 -> [_ w705 w713 w721 w729 w737 w745 w753 w761 w769 w777 w785 w793 w801 w809 w817 w825 w833 w841 w849 w857 w865 w873 w881 w889 w897 w905]
            frame "0", Default {
            }
            frame "a" {
              n320 = Not Equal To 0?(x=w705) -> (x != 0?=w706:bool)
              n321 = case shown="True" w706 {
                tunnel: w708 -> [w709 w712]
                tunnel: [w709 w710] -> w707
                frame False {
                }
                frame True {
                  n322 = Build Array (concatenate)(w712, "a") -> (w710:string[])
                }
              }
            }
            frame "b" {
              n323 = Not Equal To 0?(x=w713) -> (x != 0?=w716:bool)
              n324 = case shown="True" w716 {
                tunnel: w715 -> [w717 w720]
                tunnel: [w717 w718] -> w714
                frame False {
                }
                frame True {
                  n325 = Build Array (concatenate)(w720, "b") -> (w718:string[])
                }
              }
            }
            frame "c" {
              n326 = Not Equal To 0?(x=w721) -> (x != 0?=w724:bool)
              n327 = case shown="True" w724 {
                tunnel: w723 -> [w725 w728]
                tunnel: [w725 w726] -> w722
                frame False {
                }
                frame True {
                  n328 = Build Array (concatenate)(w728, "c") -> (w726:string[])
                }
              }
            }
            frame "d" {
              n329 = Not Equal To 0?(x=w729) -> (x != 0?=w732:bool)
              n330 = case shown="True" w732 {
                tunnel: w731 -> [w733 w736]
                tunnel: [w733 w734] -> w730
                frame False {
                }
                frame True {
                  n331 = Build Array (concatenate)(w736, "d") -> (w734:string[])
                }
              }
            }
            frame "e" {
              n332 = Not Equal To 0?(x=w737) -> (x != 0?=w740:bool)
              n333 = case shown="True" w740 {
                tunnel: w739 -> [w741 w744]
                tunnel: [w741 w742] -> w738
                frame False {
                }
                frame True {
                  n334 = Build Array (concatenate)(w744, "e") -> (w742:string[])
                }
              }
            }
            frame "f" {
              n335 = Not Equal To 0?(x=w745) -> (x != 0?=w748:bool)
              n336 = case shown="True" w748 {
                tunnel: w747 -> [w749 w752]
                tunnel: [w749 w750] -> w746
                frame False {
                }
                frame True {
                  n337 = Build Array (concatenate)(w752, "f") -> (w750:string[])
                }
              }
            }
            frame "g" {
              n338 = Not Equal To 0?(x=w753) -> (x != 0?=w756:bool)
              n339 = case shown="True" w756 {
                tunnel: w755 -> [w757 w760]
                tunnel: [w757 w758] -> w754
                frame False {
                }
                frame True {
                  n340 = Build Array (concatenate)(w760, "g") -> (w758:string[])
                }
              }
            }
            frame "h" {
              n341 = Not Equal To 0?(x=w761) -> (x != 0?=w764:bool)
              n342 = case shown="True" w764 {
                tunnel: w763 -> [w765 w768]
                tunnel: [w765 w766] -> w762
                frame False {
                }
                frame True {
                  n343 = Build Array (concatenate)(w768, "h") -> (w766:string[])
                }
              }
            }
            frame "i" {
              n344 = Not Equal To 0?(x=w769) -> (x != 0?=w772:bool)
              n345 = case shown="True" w772 {
                tunnel: w771 -> [w773 w776]
                tunnel: [w773 w774] -> w770
                frame False {
                }
                frame True {
                  n346 = Build Array (concatenate)(w776, "i") -> (w774:string[])
                }
              }
            }
            frame "j" {
              n347 = Not Equal To 0?(x=w777) -> (x != 0?=w780:bool)
              n348 = case shown="True" w780 {
                tunnel: w779 -> [w781 w784]
                tunnel: [w781 w782] -> w778
                frame False {
                }
                frame True {
                  n349 = Build Array (concatenate)(w784, "j") -> (w782:string[])
                }
              }
            }
            frame "k" {
              n350 = Not Equal To 0?(x=w785) -> (x != 0?=w788:bool)
              n351 = case shown="True" w788 {
                tunnel: w787 -> [w789 w792]
                tunnel: [w789 w790] -> w786
                frame False {
                }
                frame True {
                  n352 = Build Array (concatenate)(w792, "k") -> (w790:string[])
                }
              }
            }
            frame "l" {
              n353 = Not Equal To 0?(x=w793) -> (x != 0?=w796:bool)
              n354 = case shown="True" w796 {
                tunnel: w795 -> [w797 w800]
                tunnel: [w797 w798] -> w794
                frame False {
                }
                frame True {
                  n355 = Build Array (concatenate)(w800, "l") -> (w798:string[])
                }
              }
            }
            frame "m" {
              n356 = Not Equal To 0?(x=w801) -> (x != 0?=w804:bool)
              n357 = case shown="True" w804 {
                tunnel: w803 -> [w805 w808]
                tunnel: [w805 w806] -> w802
                frame False {
                }
                frame True {
                  n358 = Build Array (concatenate)(w808, "m") -> (w806:string[])
                }
              }
            }
            frame "n" {
              n359 = Not Equal To 0?(x=w809) -> (x != 0?=w812:bool)
              n360 = case shown="True" w812 {
                tunnel: w811 -> [w813 w816]
                tunnel: [w813 w814] -> w810
                frame False {
                }
                frame True {
                  n361 = Build Array (concatenate)(w816, "n") -> (w814:string[])
                }
              }
            }
            frame "o" {
              n362 = Not Equal To 0?(x=w817) -> (x != 0?=w820:bool)
              n363 = case shown="True" w820 {
                tunnel: w819 -> [w821 w824]
                tunnel: [w821 w822] -> w818
                frame False {
                }
                frame True {
                  n364 = Build Array (concatenate)(w824, "o") -> (w822:string[])
                }
              }
            }
            frame "p" {
              n365 = Not Equal To 0?(x=w825) -> (x != 0?=w828:bool)
              n366 = case shown="True" w828 {
                tunnel: w827 -> [w829 w832]
                tunnel: [w829 w830] -> w826
                frame False {
                }
                frame True {
                  n367 = Build Array (concatenate)(w832, "p") -> (w830:string[])
                }
              }
            }
            frame "q" {
              n368 = Not Equal To 0?(x=w833) -> (x != 0?=w836:bool)
              n369 = case shown="True" w836 {
                tunnel: w835 -> [w837 w840]
                tunnel: [w837 w838] -> w834
                frame False {
                }
                frame True {
                  n370 = Build Array (concatenate)(w840, "q") -> (w838:string[])
                }
              }
            }
            frame "r" {
              n371 = Not Equal To 0?(x=w841) -> (x != 0?=w844:bool)
              n372 = case shown="True" w844 {
                tunnel: w843 -> [w845 w848]
                tunnel: [w845 w846] -> w842
                frame False {
                }
                frame True {
                  n373 = Build Array (concatenate)(w848, "r") -> (w846:string[])
                }
              }
            }
            frame "s" {
              n374 = Not Equal To 0?(x=w849) -> (x != 0?=w852:bool)
              n375 = case shown="True" w852 {
                tunnel: w851 -> [w853 w856]
                tunnel: [w853 w854] -> w850
                frame False {
                }
                frame True {
                  n376 = Build Array (concatenate)(w856, "s") -> (w854:string[])
                }
              }
            }
            frame "t" {
              n377 = Not Equal To 0?(x=w857) -> (x != 0?=w860:bool)
              n378 = case shown="True" w860 {
                tunnel: w859 -> [w861 w864]
                tunnel: [w861 w862] -> w858
                frame False {
                }
                frame True {
                  n379 = Build Array (concatenate)(w864, "t") -> (w862:string[])
                }
              }
            }
            frame "u" {
              n380 = Not Equal To 0?(x=w865) -> (x != 0?=w868:bool)
              n381 = case shown="True" w868 {
                tunnel: w867 -> [w869 w872]
                tunnel: [w869 w870] -> w866
                frame False {
                }
                frame True {
                  n382 = Build Array (concatenate)(w872, "u") -> (w870:string[])
                }
              }
            }
            frame "v" {
              n383 = Not Equal To 0?(x=w873) -> (x != 0?=w876:bool)
              n384 = case shown="True" w876 {
                tunnel: w875 -> [w877 w880]
                tunnel: [w877 w878] -> w874
                frame False {
                }
                frame True {
                  n385 = Build Array (concatenate)(w880, "v") -> (w878:string[])
                }
              }
            }
            frame "x" {
              n386 = Not Equal To 0?(x=w881) -> (x != 0?=w884:bool)
              n387 = case shown="True" w884 {
                tunnel: w883 -> [w885 w888]
                tunnel: [w885 w886] -> w882
                frame False {
                }
                frame True {
                  n388 = Build Array (concatenate)(w888, "x") -> (w886:string[])
                }
              }
            }
            frame "y" {
              n389 = Not Equal To 0?(x=w889) -> (x != 0?=w892:bool)
              n390 = case shown="True" w892 {
                tunnel: w891 -> [w893 w896]
                tunnel: [w893 w894] -> w890
                frame False {
                }
                frame True {
                  n391 = Build Array (concatenate)(w896, "y") -> (w894:string[])
                }
              }
            }
            frame "w" {
              n392 = Not Equal To 0?(x=w897) -> (x != 0?=w900:bool)
              n393 = case shown="True" w900 {
                tunnel: w899 -> [w901 w904]
                tunnel: [w901 w902] -> w898
                frame False {
                }
                frame True {
                  n394 = Build Array (concatenate)(w904, "w") -> (w902:string[])
                }
              }
            }
            frame "z" {
              n395 = Not Equal To 0?(x=w905) -> (x != 0?=w908:bool)
              n396 = case shown="True" w908 {
                tunnel: w907 -> [w909 w912]
                tunnel: [w909 w910] -> w906
                frame False {
                }
                frame True {
                  n397 = Build Array (concatenate)(w912, "z") -> (w910:string[])
                }
              }
            }
          }
          n398 = Equal?(x=w700, y=w697) -> (x = y?=w699:bool)
        }
      }
    }
  }
  "Array 2" <- w1
